vi "Save_to_Project.vi"(8 "error in (no error)":errorcluster, 9 "index in":string, 10 "buildObject":T1, 11 "IB_RegDest_Label in":refnum<class "IB_RegDest_Label.lvclass">) -> (0 "error out":errorcluster, 1 "index out":string, 2 "buildObject out":T1, 3 "IB_RegDest_Label out":refnum<class "IB_RegDest_Label.lvclass">, 5 "saved?":bool)   [LabVIEW 2020, in "IB_RegDest_Label.lvclass"]
uses:
  <vilib>/AppBuilder/IB_Classes/RegDest/RegDest_Label/IB_RegDest_Label.lvclass
  <vilib>/AppBuilder/IB_Classes/RegDest/RegDest_Label/IB_RegDest_Label.lvclass/IB_RegDest_Label.ctl
  <resource>/Framework/Providers/API/ItemRef.ctl
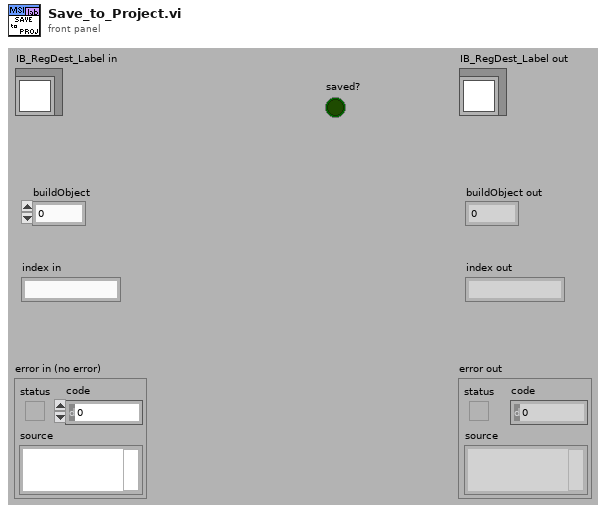
[diagram p1: front panel]
types:
  T1 = typedef "ItemRef.ctl" = u64
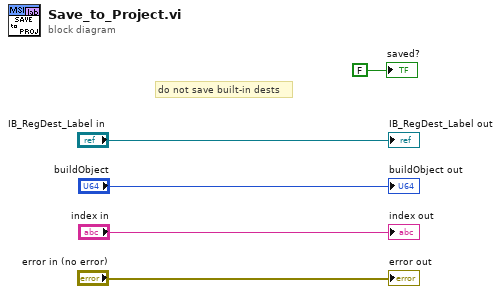
[diagram p0: block diagram]
diagram:
  # "do not save built-in dests"
  "error out" <- "error in (no error)"
  "IB_RegDest_Label out" <- "IB_RegDest_Label in"
  "buildObject out" <- "buildObject"
  "index out" <- "index in"
  "saved?" <- FALSE ("saved?")
